vi "Robot Main.vi"() -> ()   [LabVIEW 2013]
doc: "This VI imlements the framework and scheduler for your robotics program. It should not be necessary to modify the framework. You are expected to add your code to the VIs called from Robot Main, the ones located in the Team Code within the project."
uses:
  <vilib>/Rock Robotics/WPI/Camera/WPI_CameraImageSize.ctl
  <vilib>/Rock Robotics/WPI/DriverStation/WPI_DriverStationRobotMode2.ctl
  Robot Global Data.vi
panel:
  out "Application:Version Number":string
  out "Library:Version":T1
  out "Robot Mode":T2
  out "Timings":cluster{"Call Name":string, "Delta (ms)":u32}[](array[cluster])
  in  "milliseconds to wait":u32
  in  "Image Size":T3=enum."320x240"
  in  "Enable Vision":bool
  in  "Finish":bool
  # "Assign Proper Solenoid to Blocker"
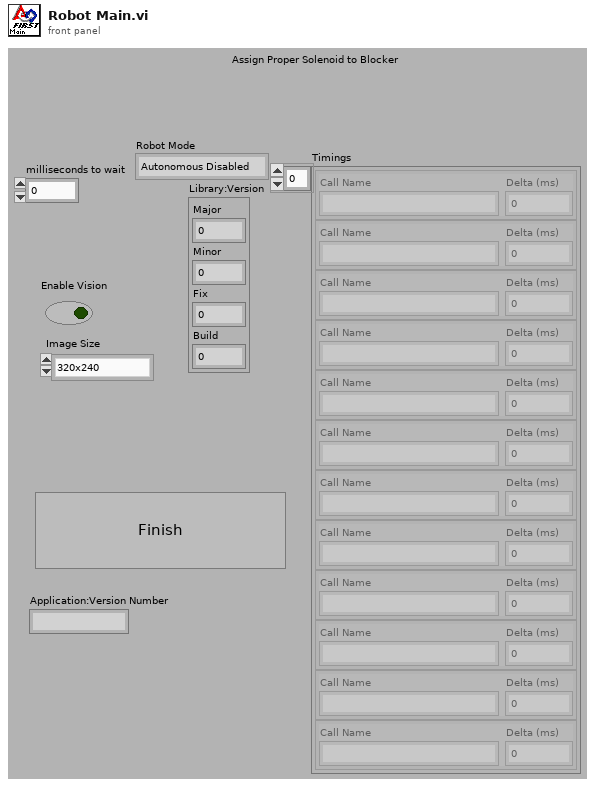
[diagram p1: front panel]
types:
  T1 = cluster{"Major":u16, "Minor":u16, "Fix":u16, "Build":u16}
  T2 = typedef "WPI_DriverStationRobotMode2.ctl" = enum16{"Autonomous Disabled", "Autonomous Enabled", "Teleop Disabled", "Teleop Enabled", "Timeout", "Finish", "Test Disabled", "Test Enabled"}
  T3 = typedef "WPI_CameraImageSize.ctl" = enum16{"640x480", "320x240", "160x120"}
  T4 = typedef "WPI_DriverStationMatch Info.ctl" = cluster{"Autonomous Elapsed Seconds":dbl, "TeleOp Elapsed Seconds":dbl, "Disabled Elapsed Seconds":dbl, "Visited Autonomous":bool, "Visited TeleOp":bool, "Visited Disabled":bool, "Autonomous Settings":cluster{"Autonomous Style":enum16{"Iterative", "Independent"}, "VI Refnum":refnum<vi>}}
  T5 = typedef "WPI_DriverStationDerivedRobotMode.ctl" = enum16{"Init", "Execute", "Stop"}
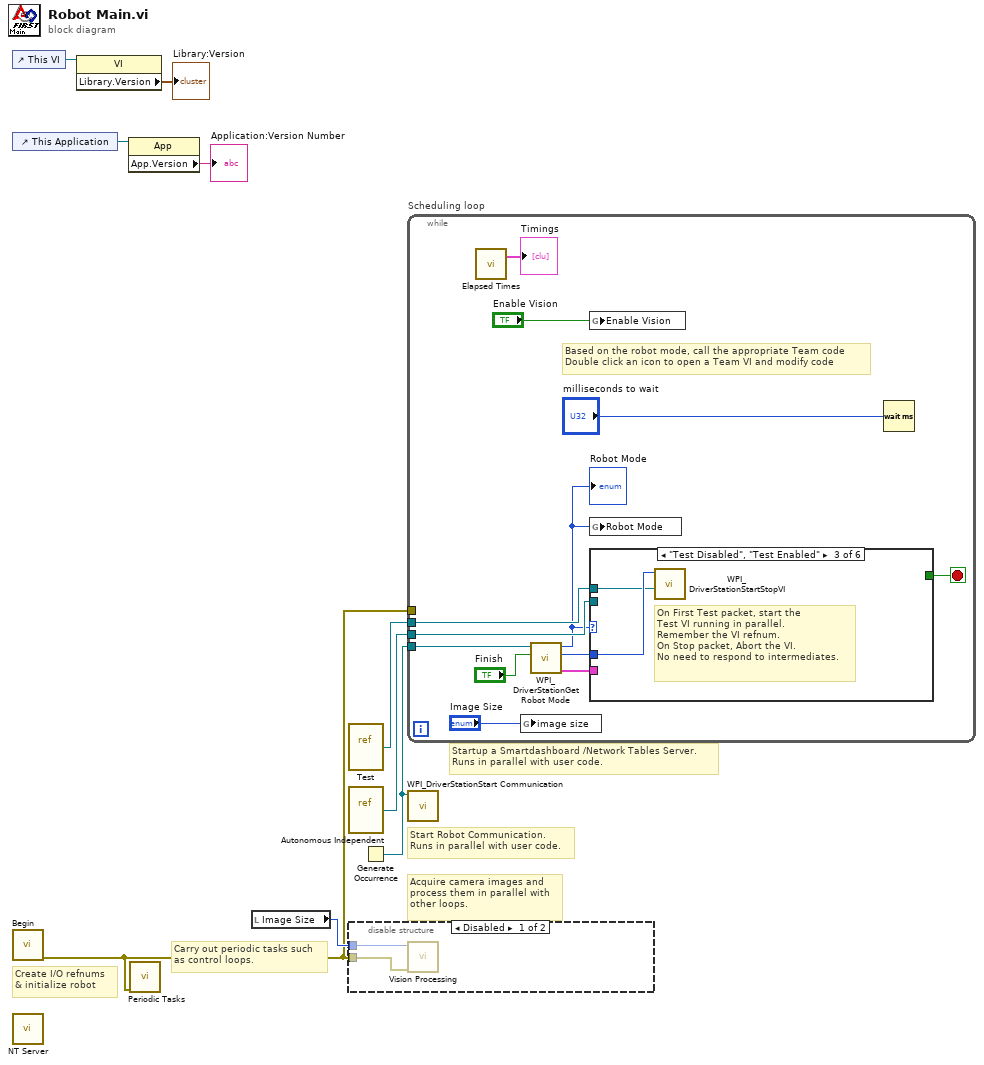
[diagram p0: block diagram]
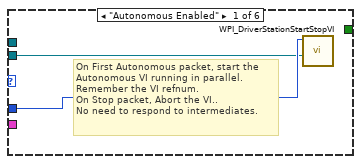
[diagram p3: hidden frame]
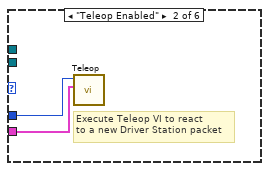
[diagram p4: hidden frame]
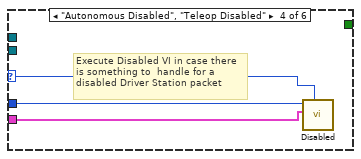
[diagram p5: hidden frame]
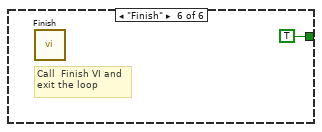
[diagram p7: hidden frame]
diagram:
  # "Startup a Smartdashboard /Network Tables Server.\nRuns in parallel with user code."
  # "Carry out periodic tasks such\nas control loops."
  # "Acquire camera images and\nprocess them in parallel with\nother loops."
  # "Create I/O refnums\n& initialize robot"
  # "Start Robot Communication.\nRuns in parallel with user code."
  n1 = control-ref of="This VI"() -> (w4:refnum<vi>)
  n2 = control-ref of="This Application"() -> (w5:refnum<vi>)
  n3 = call "Begin.vi"() -> ("error out"=w1:errorcluster)  [unwired: 1 in, 10 out]
  n4 = call <vilib>:"NT Server.vi"() -> ()  [unwired: 12 in]
  n5 = property class="VI"(reference=w4) -> ("Library.Version"=→"Library:Version":T1)  [unwired: 1 in, 2 out]
  n6 = property class="App"(reference=w5) -> ("App.Version"=→"Application:Version Number":string)  [unwired: 1 in, 2 out]
  n7 = call "Periodic Tasks.vi"("error in"=w1) -> ()  [unwired: 1 in, 10 out]
  n8 = local read "Image Size"() -> (w6:T3)
  n9 = vi-ref "Test.vi"() -> (w7:refnum<vi>)
  n10 = vi-ref "Autonomous Independent.vi"() -> (w8:refnum<vi>)
  n11 = disable-structure shown="Disabled" {
    disable-tunnel: w1 -> [w11 _]
    disable-tunnel: w6 -> [w10 _]
    frame Disabled {
      n12 = call "Vision Processing.vi"("error in (no error)"=w11, "Image Size"=w10) -> ()  [unwired: 6 out]
    }
    frame Enabled {
    }
  }
  n13 = Generate Occurrence() -> (w9:refnum<k4>)
  n14 = while "Scheduling loop" {
    tunnel: w9 -> [w22]
    tunnel: w1 -> [_]
    tunnel: w8 -> [w17]
    tunnel: w7 -> [w15]
    stop <- w19 stop-if-true
    # "Based on the robot mode, call the appropriate Team code\nDouble click an icon to open a Team VI and modify code"
    n15 = call "Elapsed Times.vi"() -> ("Timings"=→"Timings":cluster{"Call Name":string, "Delta (ms)":u32}[])  [unwired: 3 in]
    n16 = global write "Robot Global Data.vi" "image size"("Image Size") -> ()
    n17 = call <vilib>:"WPI_DriverStationGet Robot Mode.vi"("Finish"="Finish", "DS Occurrence"=w22) -> ("Match Info out"=w20:T4, "Call Context"=w23:T5, "Robot Mode"=w14:T2)  [unwired: 7 out]
    "Robot Mode" <- w14
    n18 = global write "Robot Global Data.vi" "Enable Vision"("Enable Vision") -> ()
    n19 = global write "Robot Global Data.vi" "Robot Mode"(w14) -> ()
    n20 = case shown="\"Test Disabled\", \"Test Enabled\"" w14 {
      selector: w14 -> [_ _ _ w30 _ _]
      tunnel: w23 -> [w25 w27 w29 w32 _ _]
      tunnel: w20 -> [_ w26 _ w31 _ _]
      tunnel: [_ _ _ _ _ TRUE] -> w19
      tunnel: w17 -> [w24 _ _ _ _ _]
      tunnel: w15 -> [_ _ w28 _ _ _]
      frame "Autonomous Enabled" {
        # "On First Autonomous packet, start the\nAutonomous VI running in parallel.\nRemember the VI refnum.\nOn Stop packet, Abort the VI..\nNo need to respond to intermediates."
        n21 = call <vilib>:"WPI_DriverStationStartStopVI.vi"("VI in"=w24, "Call Context"=w25) -> ()  [unwired: 10 in]
      }
      frame "Teleop Enabled" {
        # "Execute Teleop VI to react\nto a new Driver Station packet"
        n22 = call "Teleop.vi"("Match Info"=w26, "Call Context"=w27) -> ()  [unwired: 1 in, 9 out]
      }
      frame "Test Disabled", "Test Enabled" {
        # "On First Test packet, start the\nTest VI running in parallel.\nRemember the VI refnum.\nOn Stop packet, Abort the VI.\nNo need to respond to intermediates."
        n23 = call <vilib>:"WPI_DriverStationStartStopVI.vi"("VI in"=w28, "Call Context"=w29) -> ()  [unwired: 10 in]
      }
      frame "Autonomous Disabled", "Teleop Disabled" {
        # "Execute Disabled VI in case there\nis something to  handle for a\ndisabled Driver Station packet"
        n24 = call "Disabled.vi"("Robot Mode"=w30, "Match Info"=w31, "Call Context"=w32) -> ()  [unwired: 1 in, 8 out]
      }
      frame "Timeout" {
        # "Driver Station packet didn't arrive.\nPossibly useful for diagnostics"
      }
      frame "Finish" {
        # "Call  Finish VI and\nexit the loop"
        n25 = call "Finish.vi"() -> ()  [unwired: 1 in, 7 out]
      }
    }
    n26 = Wait (ms)(milliseconds to wait="milliseconds to wait") -> ()  [unwired: 1 out]
  }
  n27 = call <vilib>:"WPI_DriverStationStart Communication.vi"("occurrence"=w9) -> ()  [unwired: 11 out]
